vi "GetSource.vi"(6 "error in":errorcluster, 9 "Terminal in":refnum<class "Terminal.lvclass">) -> (0 "error out":errorcluster, 2 "source":refnum<class "Terminal.lvclass">, 3 "Terminal out":refnum<class "Terminal.lvclass">)   [LabVIEW 2014, in "Terminal.lvclass"]
uses:
  Terminal.lvclass
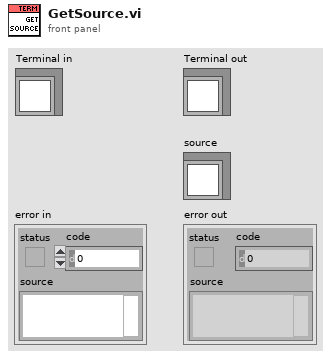
[diagram p1: front panel]
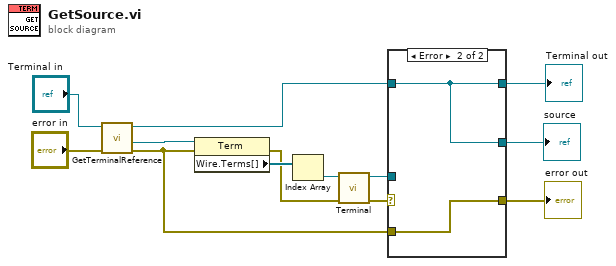
[diagram p0: block diagram]
diagram:
  n1 = call "GetTerminalReference.vi"("error in"="error in", "Terminal in"="Terminal in") -> ("error out"=w6:errorcluster, "reference"=w8:refnum<vi>, "Terminal out"=w4:refnum<class "Terminal.lvclass">)  [unwired: 7 in]
  n2 = property class="Term"(reference=w8, error in=w6) -> (error out=w11:errorcluster, "Wire.Terms[]"=w13:refnum<vi>[])  [unwired: 1 out]
  n3 = Index Array(array=w13) -> (element=w12:refnum<vi>)  [unwired: 1 in]
  n4 = call "Terminal.vi"("error in"=w11, "refnum"=w12) -> ("error out"=w7:errorcluster, "terminal"=w3:refnum<class "Terminal.lvclass">)  [unwired: 8 in]
  n5 = case shown="Error" w7 {
    selector: w7 -> [w14 _]
    tunnel: w6 -> [_ w17]
    tunnel: [w16 w18] -> w5
    tunnel: w4 -> [w16 w18]
    tunnel: w3 -> [w15 _]
    tunnel: [w15 w18] -> w2
    tunnel: [w14 w17] -> w1
    frame No Error {
    }
    frame Error {
    }
  }
  "error out" <- w1
  "Terminal out" <- w5
  "source" <- w2
